vi "Main.vi"() -> ()   [LabVIEW 2026]
uses:
  conveyorstatemachine.ctl
  colour-radio-buton.ctl
  <vilib>/numeric/Random Number (Range) DBL.vi
panel:
  out "RPM x1000":dbl(knob) scale=0.0..10.0
  out "EMERGENCY":bool
  out "Thermometer":dbl(slide)=23.333118044200546 scale=0.0..200.0
  out "emergency":bool
  out "running":bool
  out "ready":bool
  out "int":bool=TRUE
  out "state":T1
  in  "Product":u16=50
  in  "speed":i32(listbox)=2
  in  "stop":bool
  in  "Machine start":bool
  in  "COLOUR":T2=enum."colorless"
  out "Colorless prodcts":u16
  out "Grren products":u16
  out "Blue products":u16
  out "Red products":u16
  in  "Cluster":T3
  # "STATE"
  # "TEMPERATURE"
  # "RPM x1000"
  # "CONTROL"
  # "MACHINE PARAMETERS"
  # "SPEED"
  # "PRODUCTS"
  # "RPM X1000"
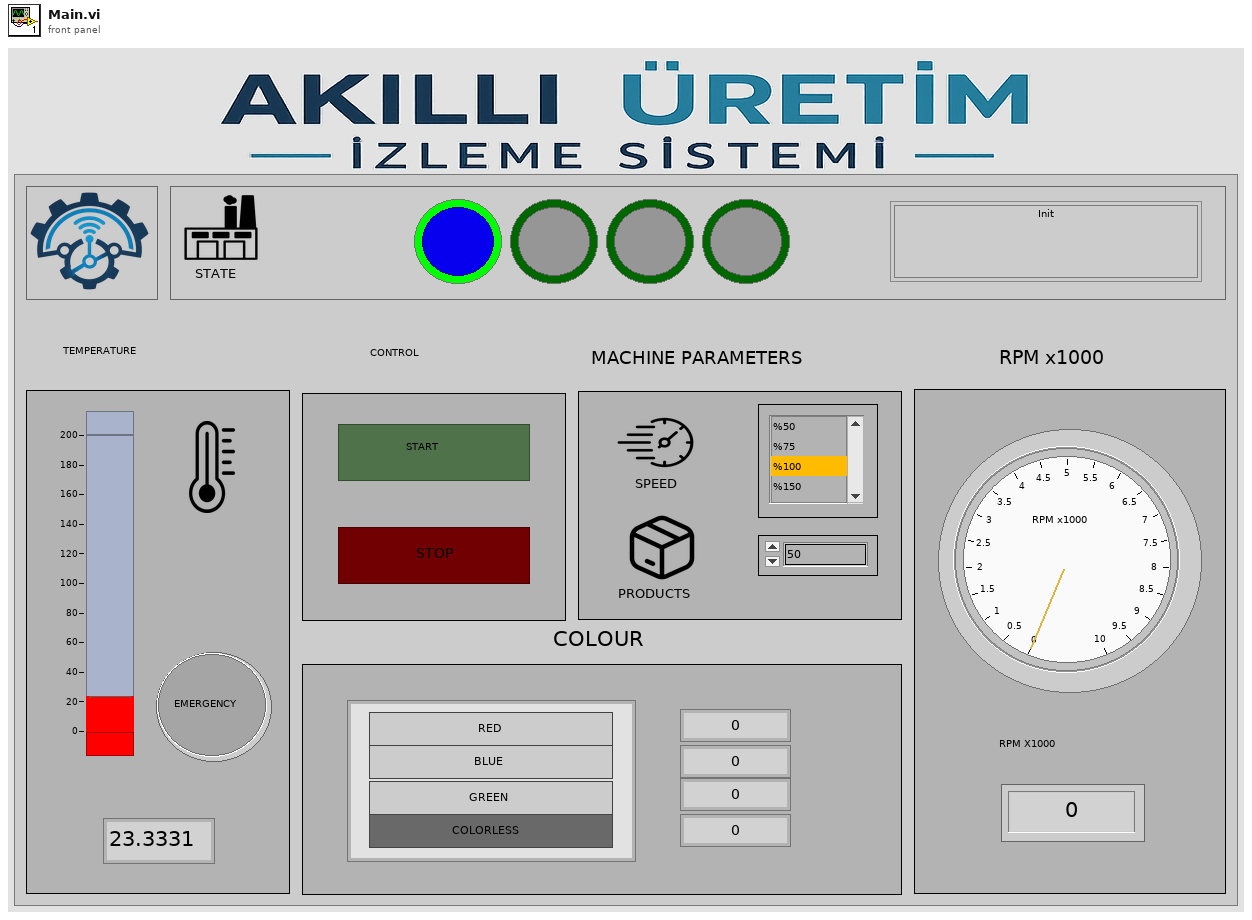
[diagram p1: front panel]
types:
  T1 = typedef "conveyorstatemachine.ctl" = enum16{"Init", "Ready", "Running", "Emergency"}
  T2 = typedef "colour-radio-buton.ctl" = enum32{"RED", "BLUE", "GREEN", "colorless"}
  T3 = cluster{"Red products":u16, "Blue products":u16, "Grren products":u16, "Colorless prodcts":u16, "Product":u16}
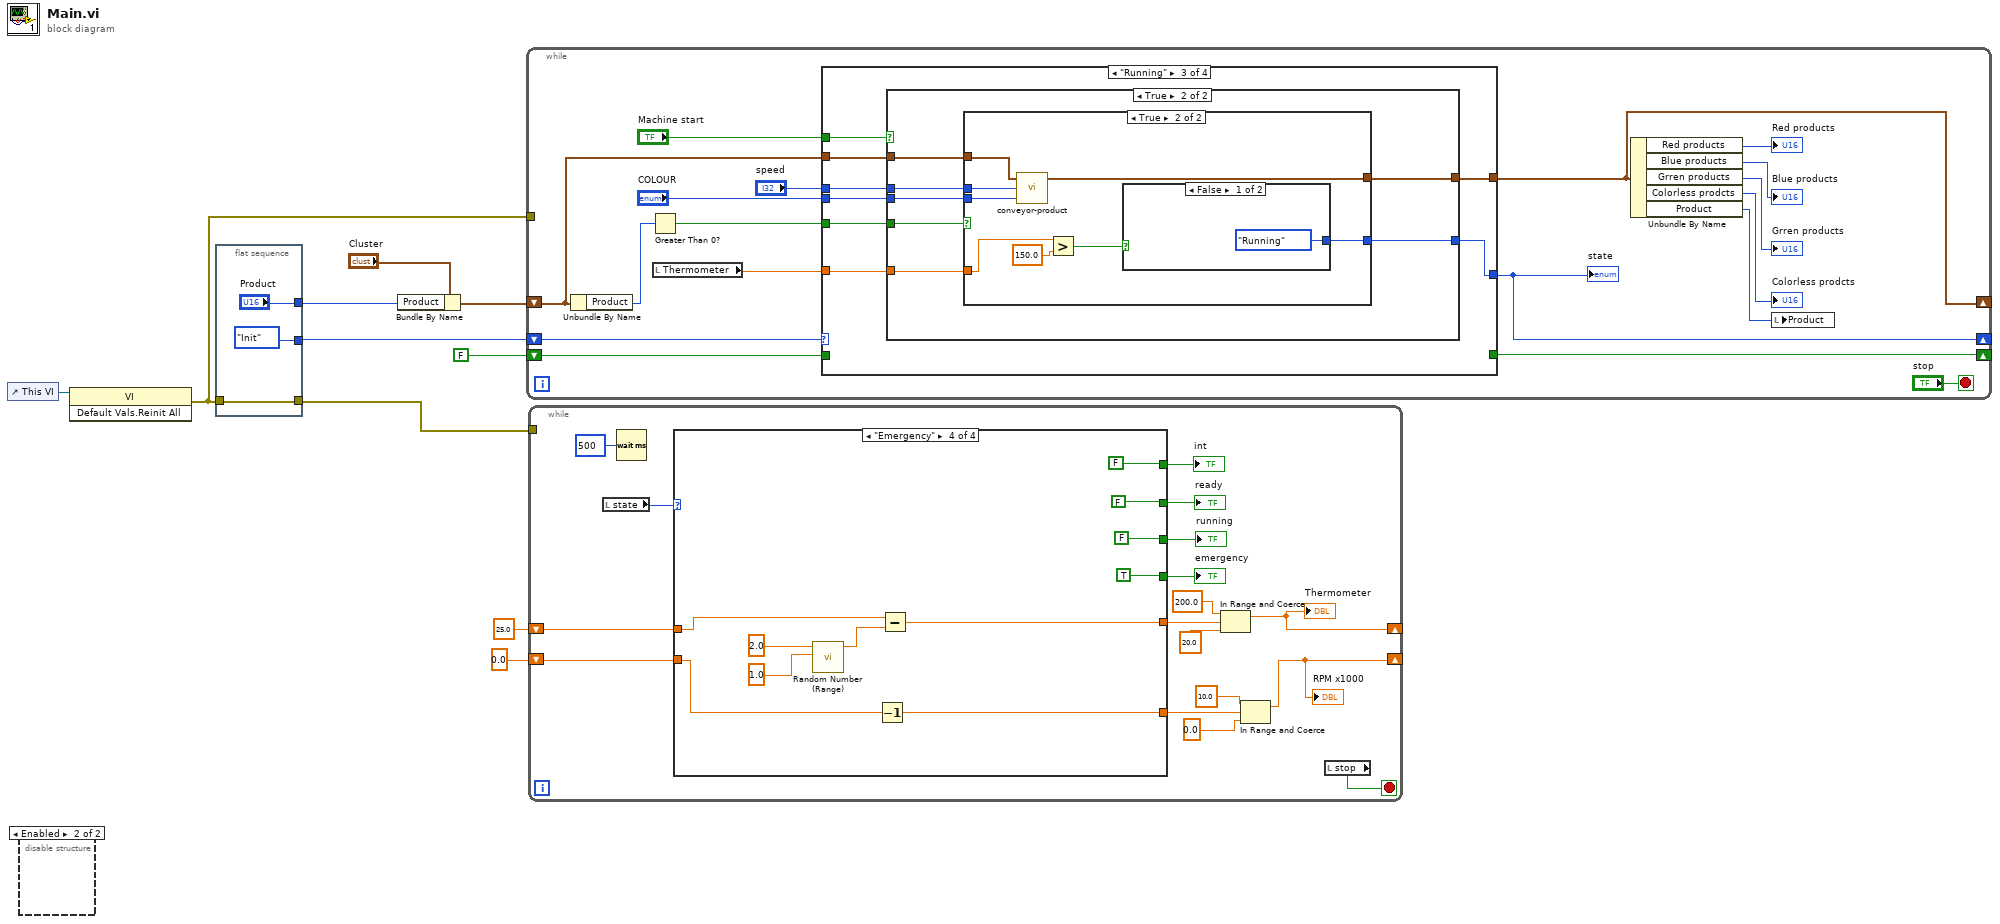
[diagram p0: block diagram]
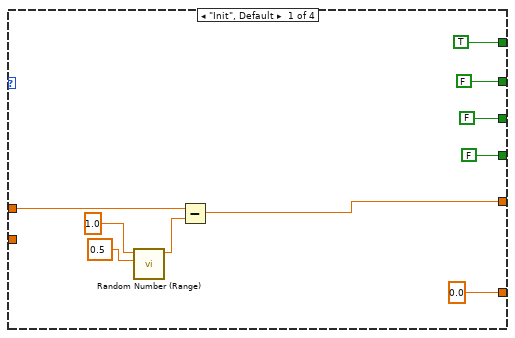
[diagram p2: hidden frame]
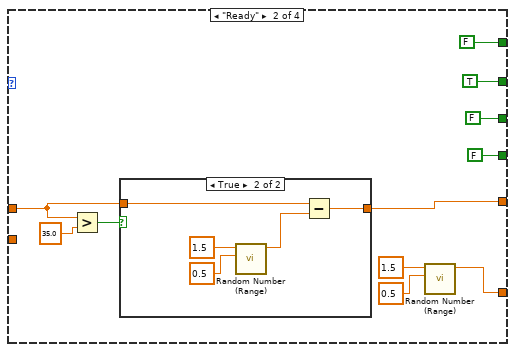
[diagram p3: hidden frame]
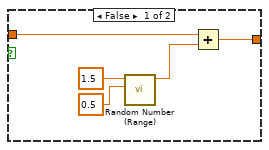
[diagram p4: hidden frame]
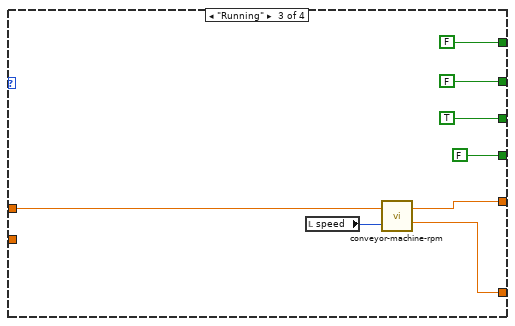
[diagram p5: hidden frame]
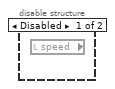
[diagram p6: hidden frame]
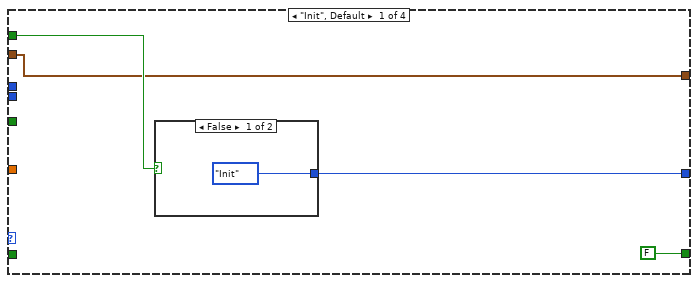
[diagram p7: hidden frame]
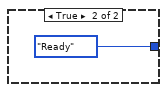
[diagram p8: hidden frame]
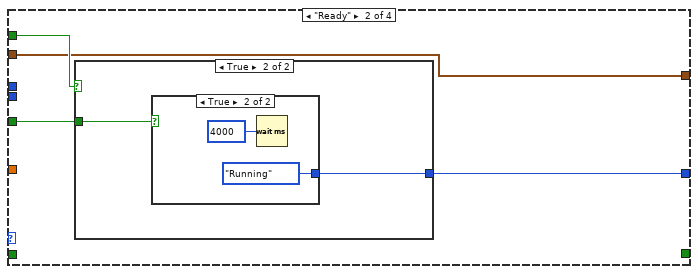
[diagram p9: hidden frame]
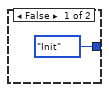
[diagram p10: hidden frame]
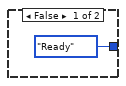
[diagram p11: hidden frame]
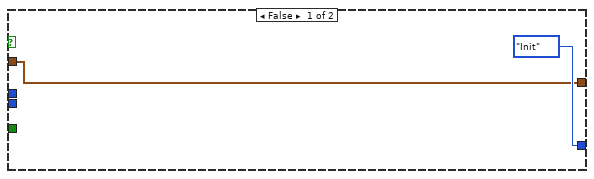
[diagram p12: hidden frame]
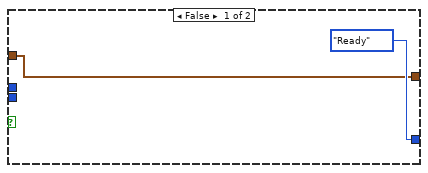
[diagram p13: hidden frame]
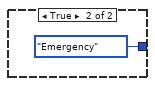
[diagram p14: hidden frame]
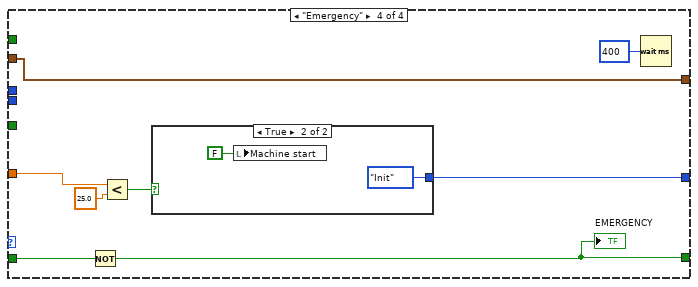
[diagram p15: hidden frame]
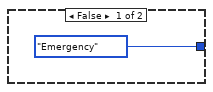
[diagram p16: hidden frame]
diagram:
  n1 = control-ref of="This VI"() -> (w5:refnum<vi>)
  n2 = disable-structure shown="Enabled" {
    frame Disabled {
      n3 = local read "speed"() -> ()  [unwired: 1 out]
    }
    frame Enabled {
    }
  }
  n4 = invoke class="VI" method="Default Vals.Reinit All"(reference=w5) -> (error out=w2:errorcluster)  [unwired: 2 in, 2 out]
  n5 = flat-sequence {
    tunnel: w2 -> [w11]
    tunnel: ["Product"] -> w4
    tunnel: [conveyorstatemachine."Init" ("state")] -> w3
    tunnel: [w11] -> w1
    frame #0 {
    }
  }
  n6 = Bundle By Name(cluster="Cluster", "Product"=w4) -> (w10:T3)
  n7 = while {
    shift-right: [w28] -> _
    shift-left: w3 -> [w27]
    shift-right: [w23] -> _
    shift-left: w10 -> [w24]
    shift-right: [w15] -> _
    shift-left: FALSE -> [w14]
    tunnel: w2 -> [_]
    stop <- "stop" stop-if-true
    n8 = Unbundle By Name(w24) -> ("Product"=w25:u16)
    n9 = Greater Than 0?(x=w25) -> (x > 0?=w29:bool)
    n10 = local read "Thermometer"() -> (w16:dbl)
    n11 = case shown="\"Running\"" w27 {
      tunnel: "Machine start" -> [w35 w41 w49 _]
      tunnel: w29 -> [_ w40 w55 _]
      tunnel: [w34 w39 w54 w80] -> w28
      tunnel: "speed" -> [_ _ w53 _]
      tunnel: w24 -> [w33 w38 w52 w84]
      tunnel: "COLOUR" -> [_ _ w51 _]
      tunnel: [w33 w38 w50 w84] -> w23
      tunnel: w16 -> [_ _ w48 w83]
      tunnel: [FALSE _ _ w78] -> w15
      tunnel: w14 -> [_ _ _ w79]
      frame "Init", Default {
        n12 = case shown="False" w35 {
          tunnel: [conveyorstatemachine."Init" ("state") conveyorstatemachine."Ready" ("state")] -> w34
          frame False {
          }
          frame True {
          }
        }
      }
      frame "Ready" {
        n13 = case shown="True" w41 {
          tunnel: w40 -> [_ w44]
          tunnel: [conveyorstatemachine."Init" ("state") w43] -> w39
          frame False {
          }
          frame True {
            n14 = case shown="True" w44 {
              tunnel: [conveyorstatemachine."Ready" ("state") conveyorstatemachine."Running" ("state")] -> w43
              frame False {
              }
              frame True {
                n15 = Wait (ms)(milliseconds to wait=u32 4000) -> ()  [unwired: 1 out]
              }
            }
          }
        }
      }
      frame "Running" {
        n16 = case shown="True" w49 {
          tunnel: w55 -> [_ w64]
          tunnel: [conveyorstatemachine."Init" ("state") w63] -> w54
          tunnel: w53 -> [_ w62]
          tunnel: w52 -> [w56 w61]
          tunnel: w51 -> [_ w60]
          tunnel: [w56 w59] -> w50
          tunnel: w48 -> [_ w58]
          frame False {
          }
          frame True {
            n17 = case shown="True" w64 {
              tunnel: [conveyorstatemachine."Ready" ("state") w68] -> w63
              tunnel: w62 -> [_ w74]
              tunnel: w61 -> [w65 w73]
              tunnel: w60 -> [_ w72]
              tunnel: [w65 w71] -> w59
              tunnel: w58 -> [_ w67]
              frame False {
              }
              frame True {
                n18 = call "conveyor-product.vi"("COLOUR"=w72, "speed in"=w74, "Cluster"=w73) -> ("Cluster o"=w71:T3)  [unwired: 2 in]
                n19 = Greater?(x=w67, y=150.0) -> (0:w70:bool)
                n20 = case shown="False" w70 {
                  tunnel: [conveyorstatemachine."Running" ("state") conveyorstatemachine."Emergency" ("state")] -> w68
                  frame False {
                  }
                  frame True {
                  }
                }
              }
            }
          }
        }
      }
      frame "Emergency" {
        n21 = Not(x=w79) -> (.not. x?=w78:bool)
        "EMERGENCY" <- w78
        n22 = Less?(x=w83, y=25.0) -> (x < y?=w81:bool)
        n23 = case shown="True" w81 {
          tunnel: [conveyorstatemachine."Emergency" ("state") conveyorstatemachine."Init" ("state")] -> w80
          frame False {
          }
          frame True {
            n24 = local write "Machine start"(FALSE ("Machine start")) -> ()
          }
        }
        n25 = Wait (ms)(milliseconds to wait=u32 400) -> ()  [unwired: 1 out]
      }
    }
    "state" <- w28
    n26 = Unbundle By Name(w23) -> ("Red products"=→"Red products":u16, "Blue products"=→"Blue products":u16, "Grren products"=→"Grren products":u16, "Colorless prodcts"=→"Colorless prodcts":u16, "Product"=w22:u16)
    n27 = local write "Product"(w22) -> ()
  }
  n28 = while {
    shift-right: [w92] -> _
    shift-left: 0.0 ("rpm out") -> [w100]
    shift-right: [w91] -> _
    shift-left: 25.0 -> [w101]
    tunnel: w1 -> [_]
    stop <- w104 stop-if-true
    n29 = local read "state"() -> (w103:T1)
    n30 = Wait (ms)(milliseconds to wait=u32 500) -> ()  [unwired: 1 out]
    n31 = case shown="\"Emergency\"" w103 {
      tunnel: [0.0 ("RPM x1000") w125 w140 w148] -> w95
      tunnel: [w110 w122 w141 w151] -> w90
      tunnel: w101 -> [w109 w121 w143 w150]
      tunnel: w100 -> [_ _ _ w149]
      tunnel: [TRUE ("int") FALSE ("int") FALSE ("int") FALSE ("int")] -> w99
      tunnel: [FALSE ("int") TRUE ("int") FALSE ("int") FALSE ("int")] -> w98
      tunnel: [FALSE ("int") FALSE ("int") TRUE ("int") FALSE ("int")] -> w97
      tunnel: [FALSE ("int") FALSE ("int") FALSE ("int") TRUE ("int")] -> w96
      frame "Init", Default {
        n32 = call-poly <vilib>:"Random Number (Range).vi"("lower bound (0)"=0.5, "upper bound (100)"=1.0) -> ("number"=w113:dbl)  [unwired: 9 in]
        n33 = Subtract(x=w109, y=w113) -> (x-y=w110:dbl)
      }
      frame "Ready" {
        n34 = Greater?(x=w121, y=35.0) -> (0:w119:bool)
        n35 = case shown="True" w119 {
          tunnel: [w126 w132] -> w122
          tunnel: w121 -> [w127 w131]
          frame False {
            n36 = call-poly <vilib>:"Random Number (Range).vi"("lower bound (0)"=0.5, "upper bound (100)"=1.5) -> ("number"=w128:dbl)  [unwired: 9 in]
            n37 = Add(x=w127, y=w128) -> (x+y=w126:dbl)
          }
          frame True {
            n38 = call-poly <vilib>:"Random Number (Range).vi"("lower bound (0)"=0.5, "upper bound (100)"=1.5) -> ("number"=w133:dbl)  [unwired: 9 in]
            n39 = Subtract(x=w131, y=w133) -> (x-y=w132:dbl)
          }
        }
        n40 = call-poly <vilib>:"Random Number (Range).vi"("lower bound (0)"=0.5, "upper bound (100)"=1.5) -> ("number"=w125:dbl)  [unwired: 9 in]
      }
      frame "Running" {
        n41 = local read "speed"() -> (w142:i32)
        n42 = call "conveyor-machine-rpm.vi"("speed in"=w142, "Temperature in"=w143) -> ("rpm out"=w140:dbl, "Temperature out"=w141:dbl)
      }
      frame "Emergency" {
        n43 = call-poly <vilib>:"Random Number (Range).vi"("lower bound (0)"=1.0, "upper bound (100)"=2.0) -> ("number"=w154:dbl)  [unwired: 9 in]
        n44 = Decrement(x=w149) -> (x-1=w148:dbl)
        n45 = Subtract(x=w150, y=w154) -> (x-y=w151:dbl)
      }
    }
    "int" <- w99
    "ready" <- w98
    "running" <- w97
    "emergency" <- w96
    n46 = In Range and Coerce(upper limit=200.0, x=w90, lower limit=20.0) -> (coerced(x)=w91:dbl)  [unwired: 1 out]
    "Thermometer" <- w91
    n47 = In Range and Coerce(upper limit=10.0, x=w95, lower limit=0.0) -> (coerced(x)=w92:dbl)  [unwired: 1 out]
    "RPM x1000" <- w92
    n48 = local read "stop"() -> (w104:bool)
  }
